vi "XML Read.vi"(8 "error in":errorcluster, 11 "XML File Path In":path) -> (0 "error out":errorcluster, 3 "FOFB Parameters":T1)   [LabVIEW 2011, in "XML VIs.lvlib"]
doc: "Reads an XML file coitaning the FOFB configuration parameters and builds a raw configuration cluster (FOFB Parameters)."
uses:
  XML VIs.lvlib
  Types Definitions/Type FOFB Parameters.ctl
  Types Definitions/Type Network Configuration.ctl
  Types Definitions/Type FA Configuration.ctl
  Types Definitions/Type Acquisition Network Configuration.ctl
  Types Definitions/Type Actuation Network Configuration.ctl
  Third Party/GXML/_subVIis/GXML SearchParser/gxml_SearchParser.vi
  Third Party/GXML/GXML.lvlib
  Type Definitions.lvlib
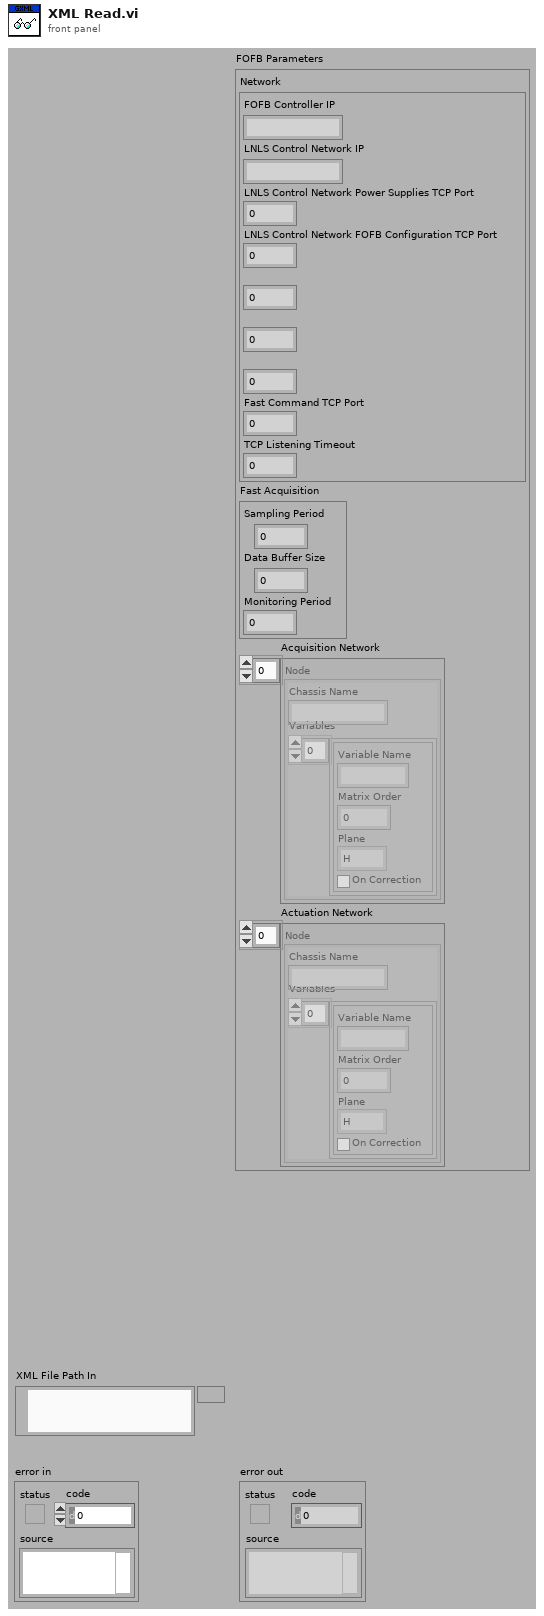
[diagram p1: front panel]
types:
  T1 = typedef "Type Definitions.lvlib/Type FOFB Parameters.ctl" = cluster{"Network":T2, "Fast Acquisition":T3, "Acquisition Network":T4, "Actuation Network":T5}
  T2 = typedef "Type Definitions.lvlib/Type Network Configuration.ctl" = cluster{"FOFB Controller IP":string, "LNLS Control Network IP":string, "LNLS Control Network Power Supplies TCP Port":u16, "LNLS Control Network FOFB Configuration TCP Port":u16, "LNLS Control Network BPMs TCP Port":u16, "Monitoring Data TCP Port":u16, "Fast Archiver TCP Port":u16, "Fast Command TCP Port":u16, "TCP Listening Timeout":i32}
  T3 = typedef "Type Definitions.lvlib/Type FA Configuration.ctl" = cluster{"Sampling Period":u32, "Data Buffer Size":u32, "Monitoring Period":u32}
  T4 = typedef "Type Definitions.lvlib/Type Acquisition Network Configuration.ctl" = cluster{"Chassis Name":string, "Variables":cluster{"Variable Name":string, "Matrix Order":u32, "Plane":enum8{"H", "V"}, "On Correction":bool}[]}[]
  T5 = typedef "Type Definitions.lvlib/Type Actuation Network Configuration.ctl" = cluster{"Chassis Name":string, "Variables":cluster{"Variable Name":string, "Matrix Order":u32, "Plane":enum8{"H", "V"}, "On Correction":bool}[]}[]
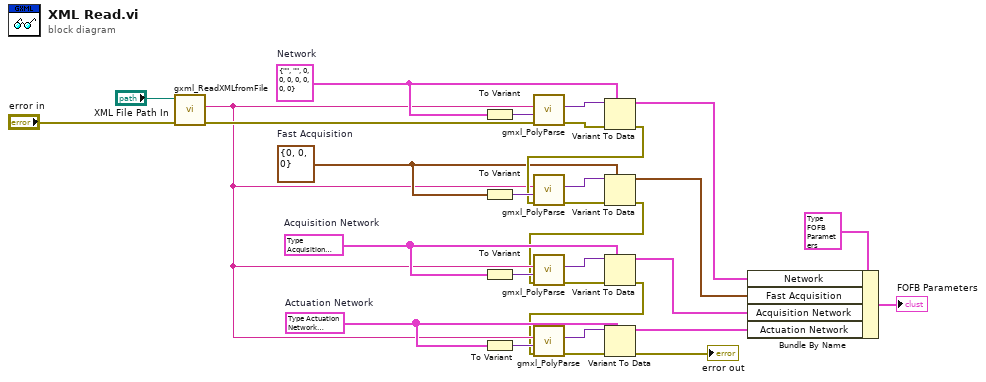
[diagram p0: block diagram]
diagram:
  w9 = T3 {"Sampling Period"=0, "Data Buffer Size"=0, "Monitoring Period"=0}  # Fast Acquisition
  w10 = T2 {"FOFB Controller IP"="", "LNLS Control Network IP"="", "LNLS Control Network Power Supplies TCP Port"=0, "LNLS Control Network FOFB Configuration TCP Port"=0, "LNLS Control Network BPMs TCP Port"=0, "Monitoring Data TCP Port"=0, "Fast Archiver TCP Port"=0, "Fast Command TCP Port"=0, "TCP Listening Timeout"=0}  # Network
  w21 = T5 [{"Chassis Name"="", "Variables"=[{"Variable Name"="", "Matrix Order"=0, "Plane"=enum."H", "On Correction"=FALSE}, {"Variable Name"="", "Matrix Order"=0, "Plane"=enum."H", "On Correction"=FALSE}, {"Variable Name"="", "Matrix Order"=0, "Plane"=enum."H", "On Correction"=FALSE}, {"Variable Name"="", "Matrix Order"=0, "Plane"=enum."H", "On Correction"=FALSE}, {"Variable Name"="", "Matrix Order"=0, "Plane"=enum."H", "On Correction"=FALSE}, {"Variable Name"="", "Matrix Order"=0, "Plane"=enum."H", "On Correction"=FALSE}, {"Variable Name"="", "Matrix Order"=0, "Plane"=enum."H", "On Correction"=FALSE}, {"Variable Name"="", "Matrix Order"=0, "Plane"=enum."H", "On Correction"=FALSE}]}]  # Actuation Network
  w22 = T4 [{"Chassis Name"="", "Variables"=[{"Variable Name"="", "Matrix Order"=0, "Plane"=enum."H", "On Correction"=FALSE}, {"Variable Name"="", "Matrix Order"=0, "Plane"=enum."H", "On Correction"=FALSE}, {"Variable Name"="", "Matrix Order"=0, "Plane"=enum."H", "On Correction"=FALSE}, {"Variable Name"="", "Matrix Order"=0, "Plane"=enum."H", "On Correction"=FALSE}, {"Variable Name"="", "Matrix Order"=0, "Plane"=enum."H", "On Correction"=FALSE}, {"Variable Name"="", "Matrix Order"=0, "Plane"=enum."H", "On Correction"=FALSE}, {"Variable Name"="", "Matrix Order"=0, "Plane"=enum."H", "On Correction"=FALSE}, {"Variable Name"="", "Matrix Order"=0, "Plane"=enum."H", "On Correction"=FALSE}]}]  # Acquisition Network
  n1 = call "gxml_ReadXMLfromFile.vi"("error in"="error in", "XML File Path"="XML File Path In") -> ("error out"=w14:errorcluster, "XML String Out"=w6:string)  [unwired: 7 in, 1 out]
  n2 = To Variant(anything=w10) -> (Variant=w15:variant)
  n3 = To Variant(anything=w9) -> (Variant=w20:variant)
  n4 = To Variant(anything=w22) -> (Variant=w29:variant)
  n5 = To Variant(anything=w21) -> (Variant=w24:variant)
  n6 = call-poly "gmxl_PolyParse.vi"("error in"=w14, "TypeDesc"=w15, "XML String In"=w6) -> ("error out"=w17:errorcluster, "Parsed Data"=w16:variant)  [unwired: 7 in]
  n7 = Variant To Data(error in=w17, type=w10, Variant=w16) -> (data=w7:T2, error out=w13:errorcluster)
  n8 = call-poly "gmxl_PolyParse.vi"("error in"=w13, "TypeDesc"=w20, "XML String In"=w6) -> ("error out"=w18:errorcluster, "Parsed Data"=w19:variant)  [unwired: 7 in]
  n9 = Variant To Data(error in=w18, type=w9, Variant=w19) -> (data=w8:T3, error out=w3:errorcluster)
  n10 = call-poly "gmxl_PolyParse.vi"("error in"=w3, "TypeDesc"=w29, "XML String In"=w6) -> ("error out"=w27:errorcluster, "Parsed Data"=w28:variant)  [unwired: 7 in]
  n11 = Variant To Data(error in=w27, type=w22, Variant=w28) -> (data=w4:T4, error out=w2:errorcluster)
  n12 = call-poly "gmxl_PolyParse.vi"("error in"=w2, "TypeDesc"=w24, "XML String In"=w6) -> ("error out"=w26:errorcluster, "Parsed Data"=w25:variant)  [unwired: 7 in]
  n13 = Variant To Data(error in=w26, type=w21, Variant=w25) -> (data=w5:T5, error out=→"error out":errorcluster)
  n14 = Bundle By Name(cluster=T1 {"Network"={"FOFB Controller IP"="", "LNLS Control Network IP"="", "LNLS Control Network Power Supplies TCP Port"=0, "LNLS Control Network FOFB Configuration TCP Port"=0, "LNLS Control Network BPMs TCP Port"=0, "Monitoring Data TCP Port"=0, "Fast Archiver TCP Port"=0, "Fast Command TCP Port"=0, "TCP Listening Timeout"=0}, "Fast Acquisition"={"Sampling Period"=0, "Data Buffer Size"=0, "Monitoring Period"=0}, "Acquisition Network"=[], "Actuation Network"=[]} ("FOFB Parameters"), "Network"=w7, "Fast Acquisition"=w8, "Acquisition Network"=w4, "Actuation Network"=w5) -> (→"FOFB Parameters":T1)
